vi "SPADQ_CalAndOffset.vi"(7 "Channel":u8, 8 "error in (no error)":errorcluster, 9 "adq_num":i32, 10 "adq_cu_ptr in":refnum<k24>, 11 "ADQAPI Ref":refnum<k24>) -> (0 "error out":errorcluster, 1 "Gain":i32, 2 "return":i32, 3 "ADQAPI Ref (out)":refnum<k24>, 4 "Offset":i32)   [LabVIEW 2022 SP3]
doc: "_____AlazarTech, Scope_____\n\nSet the Trigger delay"
uses:
  C:/Windows/System32/ADQAPI_dotNet_helper.dll
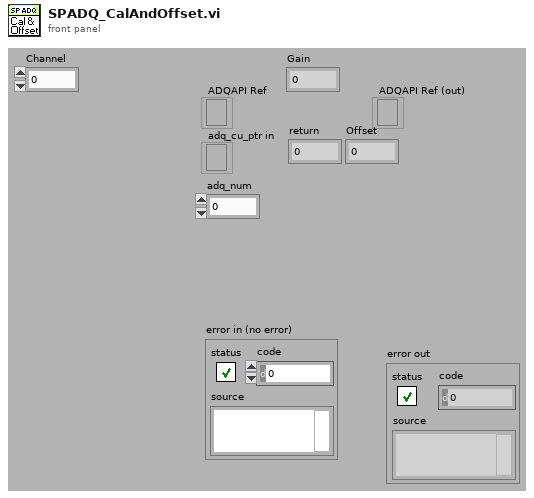
[diagram p1: front panel]
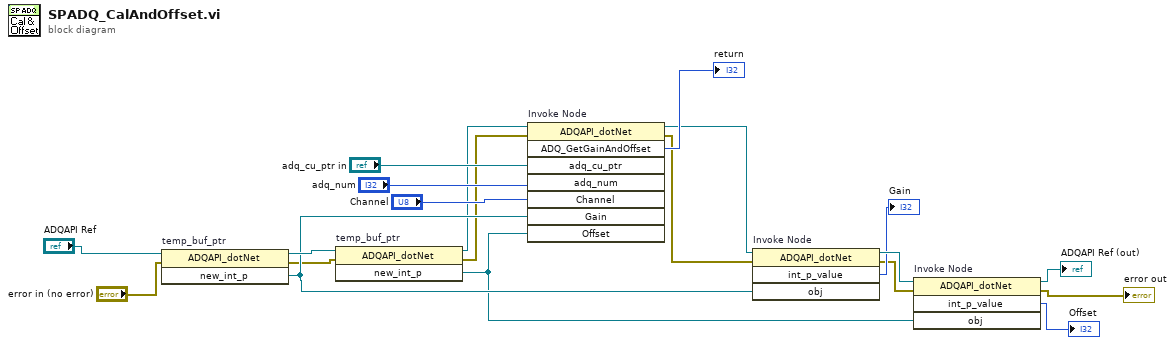
[diagram p0: block diagram]
diagram:
  n1 = invoke on="temp_buf_ptr" class="ADQAPI_dotNet" method="new_int_p"(reference="ADQAPI Ref", error in="error in (no error)") -> (reference out=w17:refnum<k24>, error out=w2:errorcluster, "new_int_p"=w16:refnum<k24>)  [unwired: 1 in]
  n2 = invoke on="temp_buf_ptr" class="ADQAPI_dotNet" method="new_int_p"(reference=w17, error in=w2) -> (reference out=w4:refnum<k24>, error out=w1:errorcluster, "new_int_p"=w15:refnum<k24>)  [unwired: 1 in]
  n3 = invoke on="Invoke Node" class="ADQAPI_dotNet" method="ADQ_GetGainAndOffset"(reference=w4, error in=w1, "adq_cu_ptr"="adq_cu_ptr in", "adq_num"="adq_num", "Channel"="Channel", "Gain"=w16, "Offset"=w15) -> (reference out=w14:refnum<k24>, error out=w7:errorcluster, "ADQ_GetGainAndOffset"=→"return":u32)  [unwired: 1 in, 5 out]
  n4 = invoke on="Invoke Node" class="ADQAPI_dotNet" method="int_p_value"(reference=w14, error in=w7, "obj"=w16) -> (reference out=w13:refnum<k24>, error out=w6:errorcluster, "int_p_value"=→"Gain":i32)  [unwired: 1 in, 1 out]
  n5 = invoke on="Invoke Node" class="ADQAPI_dotNet" method="int_p_value"(reference=w13, error in=w6, "obj"=w15) -> (reference out=→"ADQAPI Ref (out)":refnum<k24>, error out=→"error out":errorcluster, "int_p_value"=→"Offset":i32)  [unwired: 1 in, 1 out]
